vi "Configure Alarm.vi"(0 "VISA resource name":refnum<visa-resource-name>, 1 "Input Alarm Output (Disable)":u16(ring) items=["Disable", "Enable "], 2 "Input Alarm (Disable)":u16(ring) items=["Disable", "Enable"], 5 "Input Alarm Latching (Disable)":u16(ring) items=["Disable", "Enable"], 7 "Pressure Alarm Output (Disable)":u16(ring) items=["Disable", "Enable"], 9 "Pressure Alarm Latching (Disable)":u16(ring) items=["Disable", "Enable"], 11 "error in (no error)":errorcluster, 12 "Auto Increment Alarm (Disable)":u16(ring) items=["Disable", "Enable"], 13 "Auto Increment Alarm Output (Disable)":u16(ring) items=["Disable", "Enable"]) -> (4 "VISA resource name out":refnum<visa-resource-name>, 15 "error out":errorcluster)   [LabVIEW 2018, in "EFD Ultimus V.lvlib"]
doc: "Sets the options for all the Ultimus V Alarms\n\n\nHost Format: EI--INiIOoILlPOpPLbAEeAOa\ni:Enable Input Alarm (IN)\no:Enable Output of Input Alarm (IO)\nl:Latch the Input Alarm (IL)\np:Enable Output of hte Presure Alarm (PO)\nb:Latch the pressure Alarm (PL)\ne:Enable Auto Increment Alarm (AE)\na:Enable Output of hte Auto Increment Alarm (AO)"
uses:
  EFD Ultimus V.lvlib
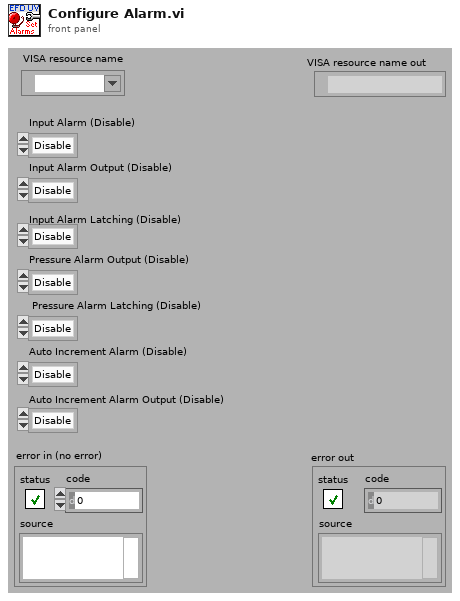
[diagram p1: front panel]
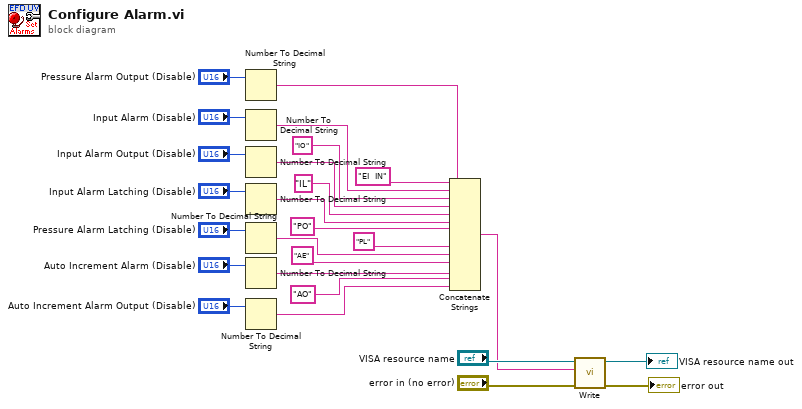
[diagram p0: block diagram]
diagram:
  n1 = Number To Decimal String(number="Pressure Alarm Output (Disable)") -> (decimal integer string=w6:string)  [unwired: 1 in]
  n2 = Number To Decimal String(number="Input Alarm (Disable)") -> (decimal integer string=w15:string)  [unwired: 1 in]
  n3 = Number To Decimal String(number="Input Alarm Output (Disable)") -> (decimal integer string=w8:string)  [unwired: 1 in]
  n4 = Number To Decimal String(number="Input Alarm Latching (Disable)") -> (decimal integer string=w7:string)  [unwired: 1 in]
  n5 = Number To Decimal String(number="Pressure Alarm Latching (Disable)") -> (decimal integer string=w5:string)  [unwired: 1 in]
  n6 = Number To Decimal String(number="Auto Increment Alarm (Disable)") -> (decimal integer string=w4:string)  [unwired: 1 in]
  n7 = Number To Decimal String(number="Auto Increment Alarm Output (Disable)") -> (decimal integer string=w3:string)  [unwired: 1 in]
  n8 = Concatenate Strings("EI  IN" ("string"), w15, "IO" ("string"), w8, "IL" ("string"), w7, "PO" ("string"), w6, "PL" ("string"), w5, "AE" ("string"), w4, "AO" ("string"), w3) -> (w17:string)
  n9 = call "Write.vi"("error in (no error)"="error in (no error)", "Command To Write"=w17, "VISA resource name"="VISA resource name") -> ("error out"=→"error out":errorcluster, "VISA resource name out"=→"VISA resource name out":refnum<visa-resource-name>)  [unwired: 7 out]
